vi "NI-XNET Main Page.vi"(8 "error in (no error)":errorcluster, 11 "Node Ptr":T2 format="%.0x") -> (0 "error out":errorcluster)   [LabVIEW 2009, in "NI-XNET Custom Device.lvlib"]
uses:
  NI-XNET Custom Device.lvlib
  <vilib>/NI VeriStand/Custom Device API/Custom Device Item Ref.ctl
  Add Outgoing.ctl
  <vilib>/NI VeriStand/Custom Device API/Get Item Property (String).vi
  <vilib>/xnet/xnet.llb/XNET String To IO Name (Cluster).vi
  <vilib>/NI VeriStand/Custom Device API/Get Item Property (Variant).vi
  <vilib>/NI VeriStand/Custom Device API/Custom Device API.lvlib
  Program Files/National Instruments/LabVIEW 2009/resource/objmgr/xnet.rc
panel:
  in  "Add outgoing":T1
  in  "Add Incoming":T1
  in  "Display Cluster Settings":bool
  in  "Header 3":cluster{"Section Name":string}={"Section Name"="Cluster Settings"}
  out "Protocol":u32(ring) items=["CAN", "FlexRay"]
  out "Comment":string
  out "Baud Rate":u32
  in  "Header 2":cluster{"Section Name":string}={"Section Name"="NI-XNET Specific Settings"}
  out "Interface":string
  out "Selected Cluster":string
  out "Database":string
  in  "Header":cluster{"Section Name":string}={"Section Name"="Custom Device Item Settings"}
  in  "Description":string
  in  "Name":string
  in  "Delete":bool
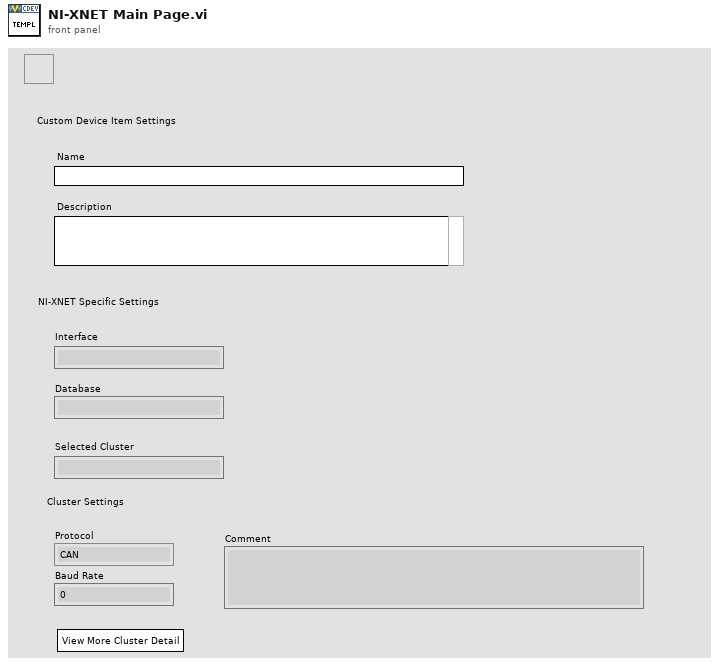
[diagram p1: front panel]
types:
  T1 = typedef "NI-XNET Custom Device.lvlib/Add Outgoing.ctl" = bool
  T2 = typedef "Custom Device API.lvlib/Custom Device Item Ref.ctl" = u64
  T3 = typedef "Custom Device API.lvlib/Custom Device Item Info.ctl" = cluster{"Name":string, "Is Channel":bool, "GUID":string}
  T4 = typedef "Custom Device API.lvlib/Custom Device Commands.ctl" = enum16{"Default", "Item renamed", "Shutdown"}
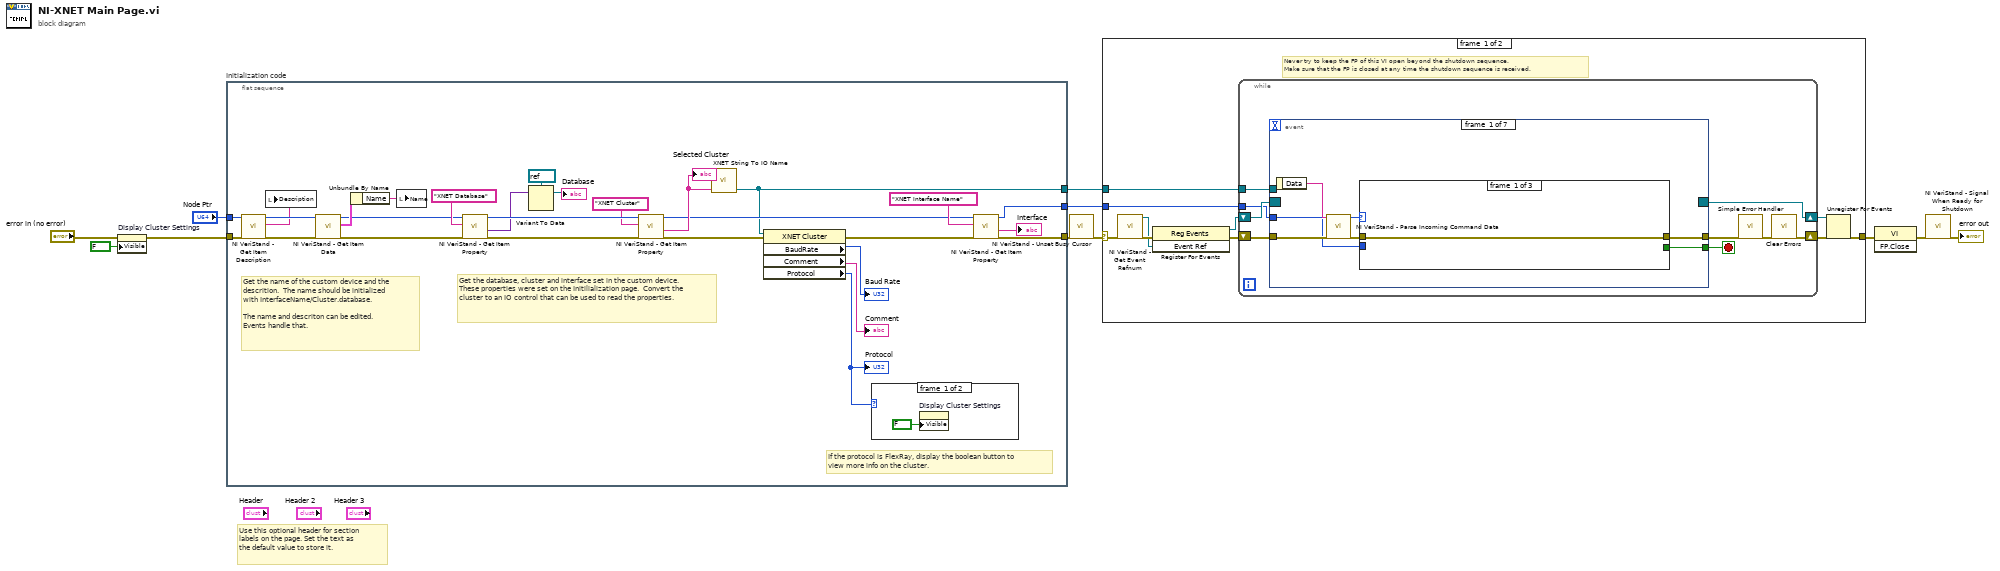
[diagram p0: block diagram]
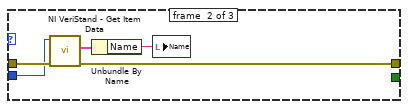
[diagram p2: hidden frame]
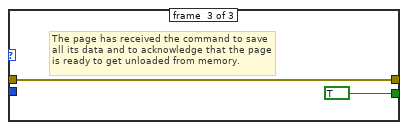
[diagram p3: hidden frame]
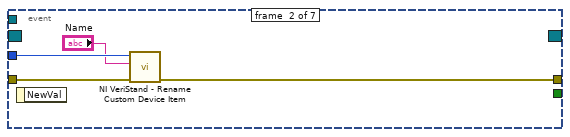
[diagram p4: hidden frame]
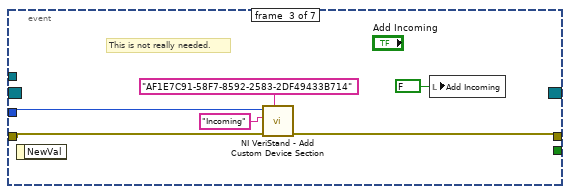
[diagram p5: hidden frame]
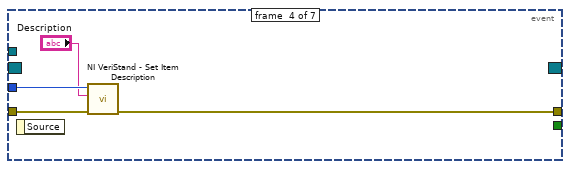
[diagram p6: hidden frame]
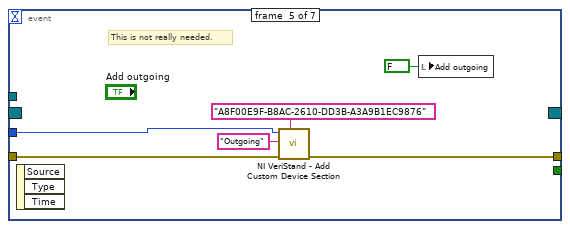
[diagram p7: hidden frame]
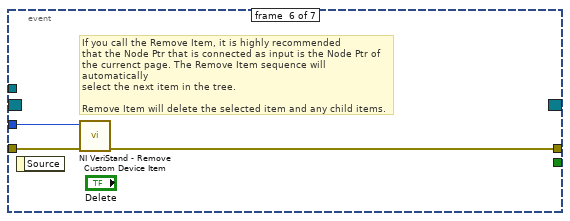
[diagram p8: hidden frame]
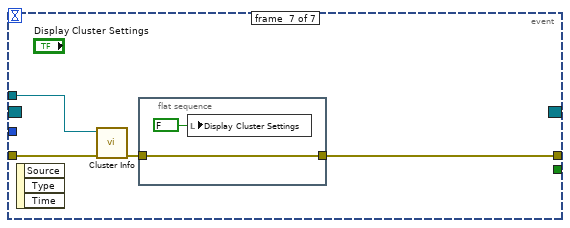
[diagram p9: hidden frame]
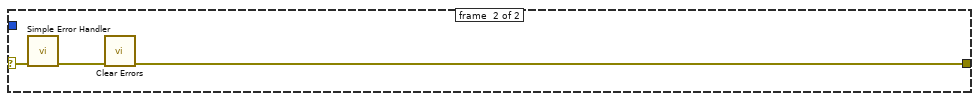
[diagram p10: hidden frame]
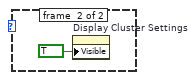
[diagram p11: hidden frame]
diagram:
  # "Use this optional header for section labels on the page. Set the text as the default value to store it."
  n1 = property on="Display Cluster Settings" class="Bool (strict)"(error in="error in (no error)", "Visible"=FALSE) -> (error out=w2:errorcluster)  [unwired: 1 in, 1 out]
  n2 = flat-sequence "Initialization code" {
    tunnel: [w28] -> w7
    tunnel: "Node Ptr" -> [w37]
    tunnel: w2 -> [w38]
    tunnel: [w20] -> w5
    tunnel: [w12] -> w1
    frame #0 {
      # "If the protocol is FlexRay, display the boolean button to view more info on the cluster."
      # "Get the database, cluster and interface set in the custom device.  These properties were set on the Initilialization page.  Convert the cluster to an IO control that can be used to read the properties."
      # "Get the name of the custom device and the descrition.  The name should be initialized with InterfaceName/Cluster.database.  \n\nThe name and descriton can be edited.  Events handle that."
      n3 = call <vilib>:"NI VeriStand - Get Item Description.vi"("error in (no error)"=w38, "Item Ref in"=w37) -> ("error out"=w35:errorcluster, "Description"=w36:string, "Item Ref out"=w39:T2)  [unwired: 7 out]
      n4 = local write "Description"(w36) -> ()
      n5 = call <vilib>:"NI VeriStand - Get Item Data.vi"("error in (no error)"=w35, "Item Ref in"=w39) -> ("error out"=w24:errorcluster, "Item Info"=w34:T3, "Item Ref out"=w23:T2)  [unwired: 7 out]
      n6 = Unbundle By Name(w34) -> ("Name"=w33:string)
      n7 = local write "Name"(w33) -> ()
      n8 = call-poly <vilib>:"NI VeriStand - Get Item Property.vi"("error in (no error)"=w24, "Property Name"="XNET Database", "Item Ref in"=w23) -> ("error out"=w21:errorcluster, "Value"=w26:variant, "Item Ref out"=w31:T2)  [unwired: 5 in, 1 out]
      n9 = Variant To Data(Variant=w26, type=refnum<k21> refnum ("XNET Database 2")) -> (data=→"Database":refnum<k21>)  [unwired: 1 in, 1 out]
      n10 = call-poly <vilib>:"NI VeriStand - Get Item Property.vi"("error in (no error)"=w21, "Property Name"="XNET Cluster", "Item Ref in"=w31) -> ("error out"=w18:errorcluster, "Value"=w19:string, "Item Ref out"=w14:T2)  [unwired: 5 in, 1 out]
      "Selected Cluster" <- w19
      n11 = call-poly <vilib>:"XNET String To IO Name.vi"("string"=w19) -> ("XNET Cluster"=w12:refnum<k21>)  [unwired: 4 in]
      n12 = property class="XNET Cluster"(reference=w12, error in=w18) -> (error out=w17:errorcluster, "BaudRate"=→"Baud Rate":u32, "Comment"=→"Comment":string, "Protocol"=w13:u32)  [unwired: 1 out]
      "Protocol" <- w13
      n13 = case shown="1" w13 {
        frame #0 {
          n14 = property on="Display Cluster Settings" class="Bool (strict)"("Visible"=FALSE) -> ()  [unwired: 2 in, 2 out]
        }
        frame #1 {
          n15 = property on="Display Cluster Settings" class="Bool (strict)"("Visible"=TRUE) -> ()  [unwired: 2 in, 2 out]
        }
      }
      n16 = call-poly <vilib>:"NI VeriStand - Get Item Property.vi"("error in (no error)"=w17, "Property Name"="XNET Interface Name", "Item Ref in"=w14) -> ("error out"=w20:errorcluster, "Value"=→"Interface":string, "Item Ref out"=w28:T2)  [unwired: 5 in, 1 out]
    }
  }
  n17 = call <vilib>:"NI VeriStand - Unset Busy Cursor.vi"("error in (no error)"=w5) -> ("error out"=w8:errorcluster)  [unwired: 10 out]
  n18 = case shown="No Error" w8 {
    selector: w8 -> [w43 w107]
    tunnel: [w48 w105] -> w11
    tunnel: w7 -> [w44 _]
    tunnel: w1 -> [w42 _]
    frame #0 {
      # "Never try to keep the FP of this VI open beyond the shutdown sequence.\nMake sure that the FP is closed at any time the shutdown sequence is received."
      n19 = call <vilib>:"NI VeriStand - Get Event Refnum.vi"("error in (no error)"=w43) -> ("error out"=w51:errorcluster, "Event Ref"=w47:refnum<user-event>)  [unwired: 9 out]
      n20 = register-events(error in=w51, w47) -> (reference out=w45:refnum<event-registration>, error out=w46:errorcluster)  [unwired: 1 in]
      n21 = while {
        tunnel: w44 -> [w56]
        shift-right: [w53] -> w49
        shift-left: w46 -> [w59]
        shift-right: [w60] -> w50
        shift-left: w45 -> [w58]
        tunnel: w42 -> [w52]
        stop <- w57 stop-if-true
        n22 = event shown="[4] \"Add outgoing\": Value Change" {
          selector: w58 -> [_ _ _ _ _ _ _]
          dyn-events: [_ _ _ _ _ _ _] -> w60
          timeout: _ -> [_ _ _ _ _ _ _]
          tunnel: w59 -> [w67 w79 w82 w88 w92 w98 w102]
          tunnel: [w63 _ _ _ _ _ _] -> w57
          tunnel: [w62 w78 w81 w87 w91 w97 w100] -> w55
          tunnel: w56 -> [w61 w77 w83 w89 w93 w96 _]
          tunnel: w52 -> [_ _ _ _ _ _ w101]
          event #0 {
            n23 = event-data() -> ("Data"=w66:string)  [unwired: 1 out]
            n24 = call <vilib>:"NI VeriStand - Parse Incoming Command Data.vi"("error in (no error)"=w67, "Data"=w66) -> ("error out"=w65:errorcluster, "Action"=w64:T4)  [unwired: 8 out]
            n25 = case shown="\"Shutdown\"" w64 {
              tunnel: w65 -> [w68 w73 w74]
              tunnel: [_ _ TRUE] -> w63
              tunnel: [w68 w70 w74] -> w62
              tunnel: w61 -> [_ w72 _]
              frame #0 {
              }
              frame #1 {
                n26 = call <vilib>:"NI VeriStand - Get Item Data.vi"("error in (no error)"=w73, "Item Ref in"=w72) -> ("error out"=w70:errorcluster, "Item Info"=w71:T3)  [unwired: 8 out]
                n27 = Unbundle By Name(w71) -> ("Name"=w69:string)
                n28 = local write "Name"(w69) -> ()
              }
              frame #2 {
                # "The page has received the command to save all its data and to acknowledge that the page is ready to get unloaded from memory."
              }
            }
          }
          event #1 {
            n29 = event-data() -> ()  [unwired: 2 out]
            n30 = call <vilib>:"NI VeriStand - Rename Custom Device Item.vi"("error in (no error)"=w79, "New Name"="Name", "Item Ref in"=w77) -> ("error out"=w78:errorcluster)  [unwired: 8 out]
          }
          event #2 {
            # "This is not really needed."
            n31 = event-data() -> ()  [unwired: 2 out]
            n32 = call <vilib>:"NI VeriStand - Add Custom Device Section.vi"("GUID (Default Section)"="AF1E7C91-58F7-8592-2583-2DF49433B714", "error in (no error)"=w82, "Section Name"="Incoming", "Parent Ref in"=w83) -> ("error out"=w81:errorcluster)  [unwired: 5 in, 2 out]
            n33 = local write "Add Incoming"(T1 FALSE ("Add Incoming")) -> ()
          }
          event #3 {
            n34 = event-data() -> ()  [unwired: 2 out]
            n35 = call <vilib>:"NI VeriStand - Set Item Description.vi"("error in (no error)"=w88, "Description"="Description", "Item Ref in"=w89) -> ("error out"=w87:errorcluster)  [unwired: 8 out]
          }
          event #4 {
            # "This is not really needed."
            n36 = event-data() -> ()  [unwired: 4 out]
            n37 = call <vilib>:"NI VeriStand - Add Custom Device Section.vi"("GUID (Default Section)"="A8F00E9F-B8AC-2610-DD3B-A3A9B1EC9876", "error in (no error)"=w92, "Section Name"="Outgoing", "Parent Ref in"=w93) -> ("error out"=w91:errorcluster)  [unwired: 5 in, 2 out]
            n38 = local write "Add outgoing"(T1 FALSE ("Add Incoming")) -> ()
          }
          event #5 {
            # "If you call the Remove Item, it is highly recommended\nthat the Node Ptr that is connected as input is the Node Ptr of\nthe currenct page. The Remove Item sequence will automatically\nselect the next item in the tree.\n\nRemove Item will delete the selected item and any child items."
            n39 = event-data() -> ()  [unwired: 2 out]
            n40 = call <vilib>:"NI VeriStand - Remove Custom Device Item.vi"("error in (no error)"=w98, "Item Ref in"=w96) -> ("error out"=w97:errorcluster)  [unwired: 1 in, 8 out]
          }
          event #6 {
            n41 = event-data() -> ()  [unwired: 4 out]
            n42 = call "Cluster Info.vi"("error in (no error)"=w102, "XNET Cluster"=w101) -> ("error out"=w99:errorcluster)  [unwired: 9 in]
            n43 = flat-sequence {
              tunnel: [w103] -> w100
              tunnel: w99 -> [w103]
              frame #0 {
                n44 = local write "Display Cluster Settings"(FALSE ("Display Cluster Settings")) -> ()
              }
            }
          }
        }
        n45 = call <vilib>:"Simple Error Handler.vi"("error in (no error)"=w55) -> ("error out"=w54:errorcluster)  [unwired: 1 in, 7 out]
        n46 = call <vilib>:"Clear Errors.vi"("error in (no error)"=w54) -> ("error out"=w53:errorcluster)  [unwired: 6 out]
      }
      n47 = Unregister For Events(event registration refnum=w50, error in=w49) -> (error out=w48:errorcluster)
    }
    frame #1 {
      n48 = call <vilib>:"Simple Error Handler.vi"("error in (no error)"=w107) -> ("error out"=w106:errorcluster)  [unwired: 1 in, 7 out]
      n49 = call <vilib>:"Clear Errors.vi"("error in (no error)"=w106) -> ("error out"=w105:errorcluster)  [unwired: 6 out]
    }
  }
  n50 = invoke class="VI" method="FP.Close"(error in=w11) -> (error out=w10:errorcluster)  [unwired: 2 in, 2 out]
  n51 = call <vilib>:"NI VeriStand - Signal When Ready for Shutdown.vi"("error in (no error)"=w10) -> ("error out"=→"error out":errorcluster)  [unwired: 10 out]
